vi "subvilijncode.vi"() -> (2 "digitaal lijn 0-1":i32[](array[numeric]), 3 "analoog lijn":dbl[](array[numeric]), 4 "stopstreep indicator":bool, 5 "lijn gedecteerd":bool)   [LabVIEW 2019]
uses:
  <vilib>/myRIO/Common/Instrument Driver Framework/Utilities/typedefs/Analog Scaling Constants.ctl
  <vilib>/myRIO/Common/Instrument Driver Framework/Utilities/typedefs/Analog Scaling Constants List.ctl
  <vilib>/myRIO/Common/Instrument Driver Framework/myRIO v1.0/AI/typedefs/AI Channels Enum.ctl
  <vilib>/myRIO/Common/Instrument Driver Framework/myRIO v1.0/AI/typedefs/AI Channels List.ctl
  <vilib>/myRIO/Common/Instrument Driver Framework/Utilities/typedefs/Generic FPGA Reference.ctl
  <vilib>/myRIO/Common/Instrument Driver Framework/Utilities/typedefs/myRIO v1.0 Reference.ctl
  <vilib>/myRIO/Common/Instrument Driver Framework/Utilities/typedefs/Hardware Version Enum.ctl
  <vilib>/myRIO/Common/Instrument Driver Framework/Utilities/typedefs/myRIO Generic Hardware Reference.ctl
  <vilib>/myRIO/Instrument Drivers/Onboard IO/AI/typedefs/AI Reference.ctl
  <vilib>/myRIO/Instrument Drivers/Onboard IO/AI/AI.lvlib
  <vilib>/myRIO/Instrument Drivers/Onboard IO/AI/vis/Read.vi
  <vilib>/userDefined/High Color/nirio_resource_hc.ctl
  <vilib>/myRIO/Common/Instrument Driver Framework/myRIO v1.0/AI/vis/myRIO v1.1 Open AI.vi
  <vilib>/myRIO/Instrument Drivers/Onboard IO/AI/vis/myRIO AI Open.xnode
  <vilib>/myRIO/Common/Instrument Driver Framework/Utilities/vis/Is FPGA Ref Available.vi
  <vilib>/myRIO/Express VI/Onboard IO/AI/AI Express VI.xnode
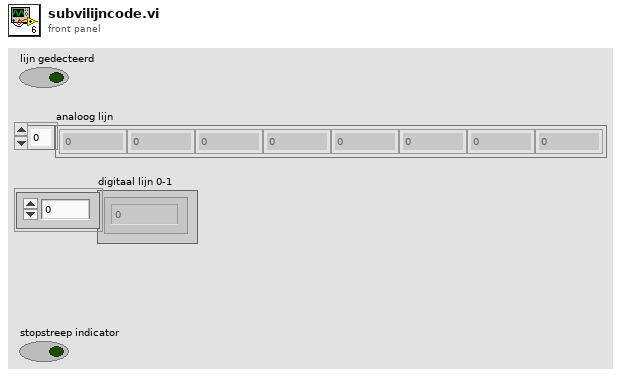
[diagram p1: front panel]
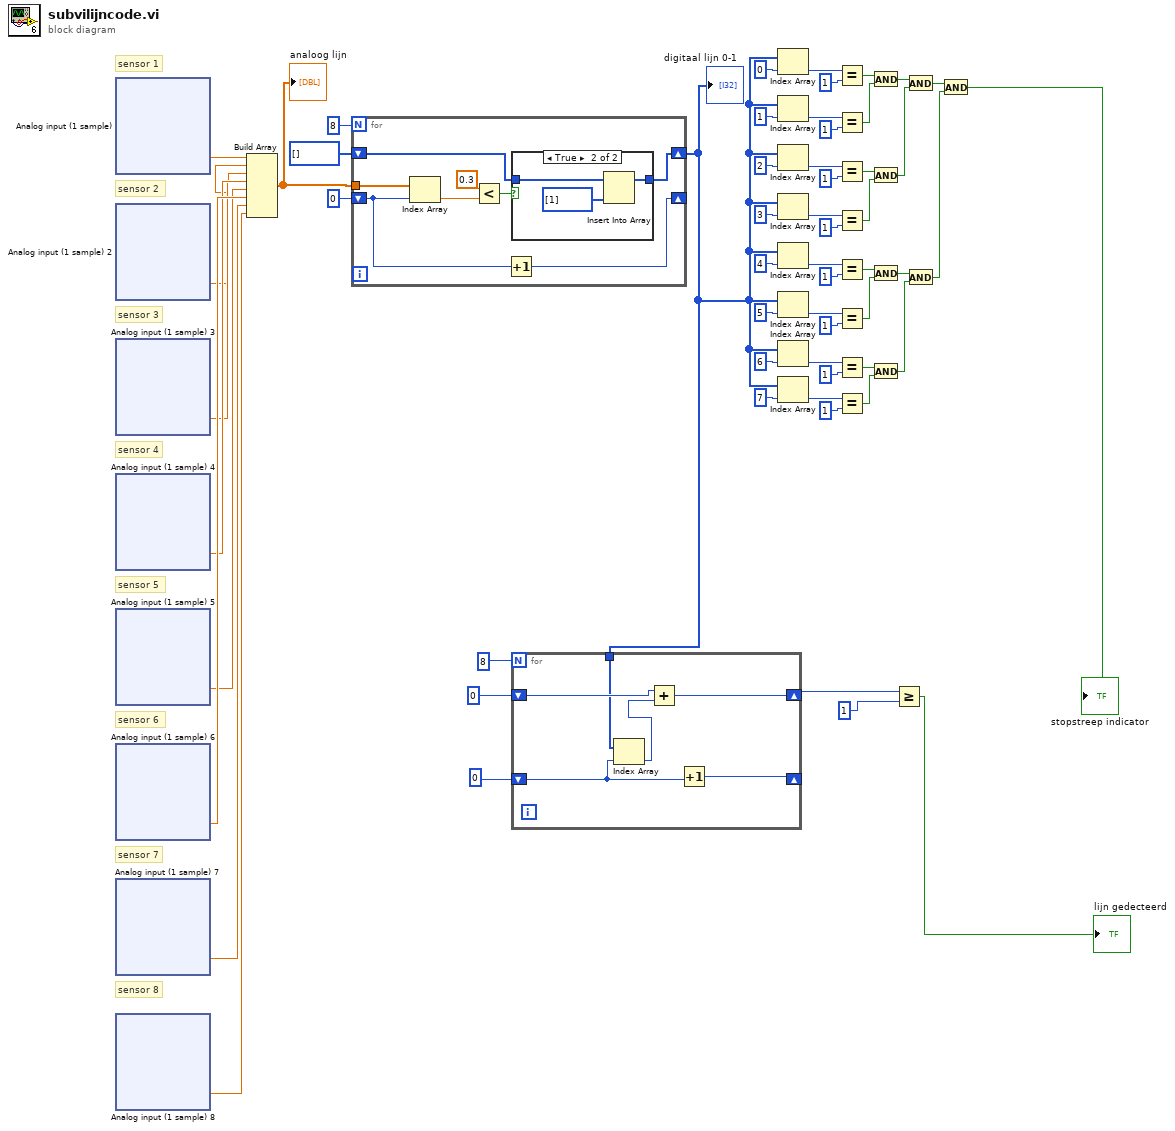
[diagram p0: block diagram]
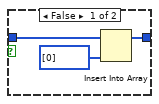
[diagram p2: hidden frame]
diagram:
  # "sensor 8"
  # "sensor 7"
  # "sensor 6"
  # "sensor 5"
  # "sensor 4"
  # "sensor 3"
  # "sensor 2"
  # "sensor 1"
  n1 = xnode "Analog input (1 sample)"() -> ("A/AI3 (Pin 9)"=w48:dbl)  [unwired: 1 in, 1 out]
  n2 = xnode "Analog input (1 sample) 2"() -> ("A/AI2 (Pin 7)"=w49:dbl)  [unwired: 1 in, 1 out]
  n3 = xnode "Analog input (1 sample) 3"() -> ("A/AI1 (Pin 5)"=w50:dbl)  [unwired: 1 in, 1 out]
  n4 = xnode "Analog input (1 sample) 4"() -> ("A/AI0 (Pin 3)"=w51:dbl)  [unwired: 1 in, 1 out]
  n5 = xnode "Analog input (1 sample) 5"() -> ("B/AI3 (Pin 9)"=w52:dbl)  [unwired: 1 in, 1 out]
  n6 = xnode "Analog input (1 sample) 6"() -> ("B/AI2 (Pin 7)"=w53:dbl)  [unwired: 1 in, 1 out]
  n7 = xnode "Analog input (1 sample) 7"() -> ("A/AI1 (Pin 5)"=w54:dbl)  [unwired: 1 in, 1 out]
  n8 = xnode "Analog input (1 sample) 8"() -> ("B/AI0 (Pin 3)"=w55:dbl)  [unwired: 1 in, 1 out]
  n9 = Build Array(w48, w49, w50, w51, w52, w53, w54, w55) -> (w56:dbl[])
  "analoog lijn" <- w56
  n10 = for {
    N: 8 -> [_]
    shift-right: [w65] -> w1
    shift-left: i32[] [] -> [w66]
    shift-right: [w63] -> _
    shift-left: 0 -> [w60]
    tunnel: w56 -> [w61]
    n11 = Index Array(array=w61, index=w60) -> (element=w62:dbl)
    n12 = Less?(x=0.3, y=w62) -> (x < y?=w64:bool)
    n13 = Increment(x=w60) -> (x+1=w63:i32)
    n14 = case shown="True" w64 {
      tunnel: w66 -> [w68 w70]
      tunnel: [w69 w72] -> w65
      frame False {
        n15 = Insert Into Array(array=w68, new element=i32[] [0]) -> (w69:i32[])  [unwired: 1 in]
      }
      frame True {
        n16 = Insert Into Array(array=w70, new element=i32[] [1]) -> (w72:i32[])  [unwired: 1 in]
      }
    }
  }
  "digitaal lijn 0-1" <- w1
  n17 = for {
    N: 8 -> [_]
    shift-right: [w78] -> _
    shift-left: 0 -> [w77]
    shift-right: [w74] -> w3
    shift-left: 0 -> [w76]
    tunnel: w1 -> [w73]
    n18 = Index Array(array=w73, index=w77) -> (element=w75:i32)
    n19 = Add(x=w76, y=w75) -> (x+y=w74:i32)
    n20 = Increment(x=w77) -> (x+1=w78:i32)
  }
  n21 = Index Array(array=w1, index=0) -> (element=w26:i32)
  n22 = Index Array(array=w1, index=1) -> (element=w47:i32)
  n23 = Index Array(array=w1, index=2) -> (element=w41:i32)
  n24 = Index Array(array=w1, index=3) -> (element=w44:i32)
  n25 = Index Array(array=w1, index=4) -> (element=w38:i32)
  n26 = Index Array(array=w1, index=5) -> (element=w35:i32)
  n27 = Index Array(array=w1, index=6) -> (element=w32:i32)
  n28 = Index Array(array=w1, index=7) -> (element=w29:i32)
  n29 = Equal?(x=w26, y=1) -> (x = y?=w23:bool)
  n30 = Equal?(x=w47, y=1) -> (x = y?=w22:bool)
  n31 = Equal?(x=w41, y=1) -> (x = y?=w21:bool)
  n32 = Equal?(x=w44, y=1) -> (x = y?=w20:bool)
  n33 = Equal?(x=w38, y=1) -> (x = y?=w19:bool)
  n34 = Equal?(x=w35, y=1) -> (x = y?=w18:bool)
  n35 = Equal?(x=w32, y=1) -> (x = y?=w17:bool)
  n36 = Equal?(x=w29, y=1) -> (x = y?=w16:bool)
  n37 = And(x=w23, y=w22) -> (x .and. y?=w15:bool)
  n38 = And(x=w21, y=w20) -> (x .and. y?=w14:bool)
  n39 = And(x=w19, y=w18) -> (x .and. y?=w13:bool)
  n40 = And(x=w17, y=w16) -> (x .and. y?=w12:bool)
  n41 = Greater Or Equal?(x=w3, y=1) -> (x >= y?=→"lijn gedecteerd":bool)
  n42 = And(x=w15, y=w14) -> (x .and. y?=w11:bool)
  n43 = And(x=w13, y=w12) -> (x .and. y?=w10:bool)
  n44 = And(x=w11, y=w10) -> (x .and. y?=→"stopstreep indicator":bool)
